vi "Refresh-selected-motor.vi"(8 "error in (no error)":errorcluster, 10 "Motor index":i32, 11 "Object ref in":T1) -> (0 "error out":errorcluster, 3 "Object ref out":T1)   [LabVIEW 2013, in "PowderDeposition.lvlib" / "PD-Main.lvclass"]
uses:
  PD-Main.lvclass
  Object-reference.ctl
  PD-Main.lvclass/PD-Main.ctl
  Write Sequence index.vi
  Write Selected motor.vi
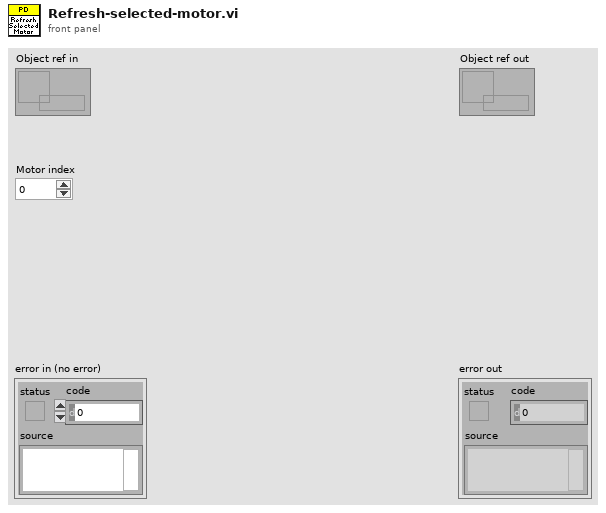
[diagram p1: front panel]
types:
  T1 = typedef "PowderDeposition.lvlib/PD-Main.lvclass/Object-reference.ctl" = refnum<data-value>
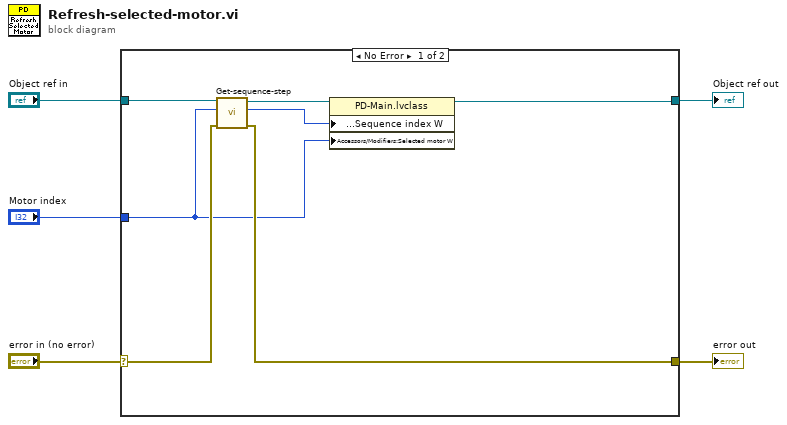
[diagram p0: block diagram]
diagram:
  n1 = case shown="No Error" "error in (no error)" {
    selector: "error in (no error)" -> [w11 w14]
    tunnel: [w8 w14] -> w4
    tunnel: [w6 w13] -> w2
    tunnel: "Object ref in" -> [w12 w13]
    tunnel: "Motor index" -> [w7 _]
    frame No Error {
      n2 = call "Get-sequence-step.vi"("error in (no error)"=w11, "Motor index"=w7, "Object ref in"=w12) -> ("error out"=w8:errorcluster, "Sequence step"=w9:i32, "Object ref out"=w10:T1)  [unwired: 6 in]
      n3 = property class="PD-Main.lvclass"(reference=w10, "Accessors/Modifiers:Sequence index W"=w9, "Accessors/Modifiers:Selected motor W"=w7) -> (reference out=w6:T1)  [unwired: 1 in, 1 out]
    }
    frame Error {
    }
  }
  "error out" <- w4
  "Object ref out" <- w2
